vi "gfitsio-get-column-type.vi"(7 "column":string, 8 "error in (no error)":errorcluster, 11 "gfits refnum":T2) -> (0 "error out":errorcluster, 1 "cfitsio datatype":T1=1 items=["ANY_HDU"=-1, "IMAGE_HDU"=0, "ASCII_TBL"=1, "BINARY_TBL"=2], 3 "dup gfits refnum":T2, 4 "variable length array?":bool)   [LabVIEW 2011, in "gfitsio.lvlib"]
doc: "Return the data type of a column in an ASCII or binary table. In the case of scaled integer columns it returns the 'equivalent' data type that is needed to store the scaled values, and not necessarily the physical data type of the unscaled values as stored in the FITS table. For example if a '1I' column in a binary table has TSCALn = 1 and TZEROn = 32768, then this column effectively contains unsigned short integer values, and thus the returned value of typecode will be TUSHORT, not TSHORT. Similarly, if a column has TTYPEn = '1I' and TSCALn = 0.12, then the returned typecode will be TFLOAT."
uses:
  gfitsio.lvlib
  gfitsio-refnum.ctl
  cfitsio-hdutypes.ctl
  gfitsio.dll
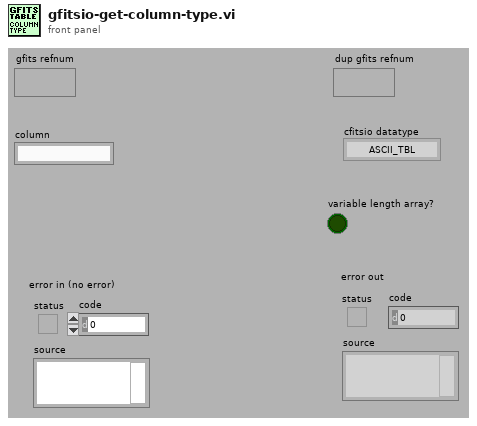
[diagram p1: front panel]
types:
  T1 = typedef "gfitsio.lvlib/cfitsio-hdutypes.ctl" = i32
  T2 = typedef "gfitsio.lvlib/gfitsio-refnum.ctl" = refnum<k1>
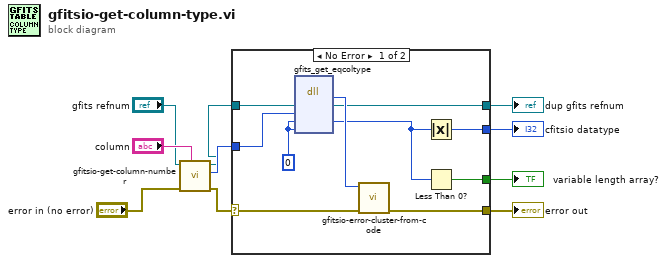
[diagram p0: block diagram]
diagram:
  n1 = call "gfitsio-get-column-number.vi"("column"="column", "error in (no error)"="error in (no error)", "gfits refnum"="gfits refnum") -> ("error out"=w4:errorcluster, "colnum"=w3:i32, "dup gfits refnum"=w1:T2)  [unwired: 6 in]
  n2 = case shown="No Error" w4 {
    selector: w4 -> [w19 w22]
    tunnel: [w18 w22] -> w10
    tunnel: w1 -> [w16 w21]
    tunnel: [w17 w21] -> w9
    tunnel: w3 -> [w15 _]
    tunnel: [w14 _] -> w8
    tunnel: [w13 _] -> w7
    frame No Error {
      w12 = 0
      n3 = dll-call lib="C:/BonOMM/BonOMM-SAOMM/SubVIs/gfitsio/gfitsio.dll" fn="gfits_get_eqcoltype"("dup gfits refnum"=w16, "colnum"=w15, "datatype"=w12, "nelements"=w12) -> (w20:i32, "dup gfits refnum"=w17:T2, "datatype"=w11:i32)  [unwired: 5 in, 2 out]
      n4 = call "gfitsio-error-cluster-from-code.vi"("error in (no error)"=w19, "error code"=w20) -> ("error out"=w18:errorcluster)  [unwired: 9 in]
      n5 = Absolute Value(x=w11) -> (abs(x)=w14:i32)
      n6 = Less Than 0?(x=w11) -> (x < 0?=w13:bool)
    }
    frame Error {
    }
  }
  "error out" <- w10
  "dup gfits refnum" <- w9
  "cfitsio datatype" <- w8
  "variable length array?" <- w7
